vi "Write Command.vi"(7 "Addr":string, 10 "Input Value":dbl, 11 "TEC Cmd":T1) -> (2 "Divisor":i32, 3 "Cmd":string)   [LabVIEW 2018, in "TE Cooler.lvlib" / "TE Cooler.lvclass"]
uses:
  TE Cooler.lvclass
  Controls/Command.ctl
  Controls/Scale IO.ctl
  Controls/Hex Cmd.ctl
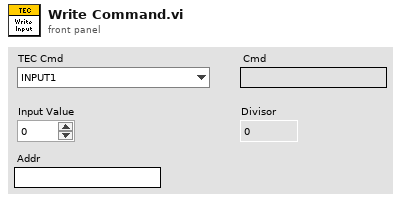
[diagram p1: front panel]
types:
  T1 = typedef "TE Cooler.lvlib/TE Cooler.lvclass/Command.ctl" = enum16{"INPUT1", "DESIRED CONTROL VALUE", "POWER OUTPUT", "ALARM STATUS", "INPUT 2", "OUTPUT CURRENT COUNTS", "ALARM TYPE", "SET TYPE DEFINE", "SENSOR TYPE", "CONTROL TYPE", "CONTROL OUTPUT POLARITY", "POWER ON/OFF", "OUTPUT SHUTDOWN IF ALARM", "FIXED DESIRED CONTROL SETTING", "PROPORTIONAL BANDWIDTH", "INTEGRAL GAIN", "DERIVATIVE GAIN", "LOW EXTERNAL SET RANGE", "HIGH EXTERNAL SET RANGE", "ALARM DEADBAND", "HIGH ALARM SETTING", "LOW ALARM SETTING", "CONTROL DEADBAND SETTING", "INPUT1 OFFSET", "INPUT2 OFFSET", "HEAT MULTIPLIER", "COOL MULTIPLIER", "OVER CURRENT COUNT COMPARE VALUE", "ALARM LATCH ENABLE", "NOT USED", "ALARM LATCH RESET", "CHOOSE SENSOR FOR ALARM FUNCTION", "CHOOSE TEMPERATURE WORKING UNITS", "EEPROM WRITE ENABLE", "OVER CURRENT CONTINUOUS", "OVER CURRENT RESTART ATTEMPTS", "JP3 DISPLAY ENABLE"}
  T2 = typedef "TE Cooler.lvlib/TE Cooler.lvclass/Hex Cmd.ctl" = string[][]
  T3 = typedef "TE Cooler.lvlib/TE Cooler.lvclass/Scale IO.ctl" = i32[][]
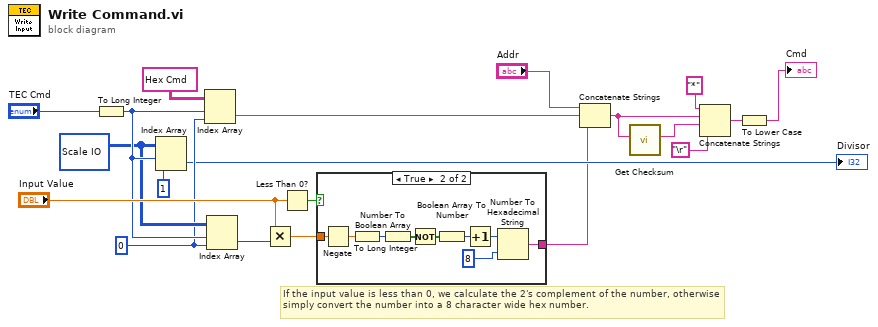
[diagram p0: block diagram]
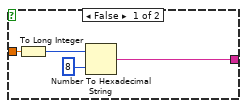
[diagram p2: hidden frame]
diagram:
  w15 = T3 [[0, 100], [0, 100], [0, 511], [0, 1], [0, 100], [0, 1], [1, 1], [1, 1], [1, 1], [1, 1], [1, 1], [1, 1], [100, 100], [100, 100], [100, 100], [100, 100], [1, 1], [1, 1], [100, 100], [100, 100], [100, 100], [100, 100], [100, 100], [100, 100], [100, 100], [100, 100], [100, 100], [1, 1], [1, 1], [0, 0], [1, 0], [1, 1], [1, 1], [1, 1], [1, 1], [1, 1], [1, 1]] ("Scale IO")
  w14 = 0 ("index (col)")
  # "If the input value is less than 0, we calculate the 2's complement of the number, otherwise simply convert the number into a 8 character wide hex number."
  n1 = To Long Integer(number="TEC Cmd") -> (32bit integer=w19:i32)
  n2 = Index Array(array=w15, index (row)=w19, index (col)=1 ("disabled index (col)")) -> (element=→"Divisor":i32)
  n3 = Index Array(array=T2 [["", "01"], ["", "03"], ["", "02"], ["", "05"], ["", "06"], ["", "07"], ["28", "41"], ["29", "42"], ["2a", "43"], ["2b", "44"], ["2c", "45"], ["2d", "46"], ["2e", "47"], ["1c", "50"], ["1d", "51"], ["1e", "52"], ["1f", "53"], ["20", "54"], ["21", "55"], ["22", "56"], ["23", "57"], ["24", "58"], ["25", "59"], ["26", "5a"], ["27", "5b"], ["0c", "5c"], ["0d", "5d"], ["0e", "5e"], ["2f", "48"], ["", ""], ["33", ""], ["31", "4a"], ["32", "4b"], ["34", "4c"], ["35", "4d"], ["0f", "5f"], ["36", "4e"]] ("Hex Cmd"), index (row)=w19, index (col)=w14) -> (element=w7:string)
  n4 = Index Array(array=w15, index (row)=w19, index (col)=w14) -> (element=w8:i32)
  n5 = Multiply(x="Input Value", y=w8) -> (x*y=w13:dbl)
  n6 = Less Than 0?(x="Input Value") -> (x < 0?=w12:bool)
  n7 = case shown="True" w12 {
    tunnel: [w23 w29] -> w2
    tunnel: w13 -> [w22 w25]
    frame False {
      n8 = To Long Integer(number=w22) -> (32bit integer=w21:i32)
      n9 = Number To Hexadecimal String(1:i16 8 ("width (-)"), 2:w21) -> (0:w23:string)
    }
    frame True {
      n10 = Negate(x=w25) -> (-x=w26:dbl)
      n11 = To Long Integer(number=w26) -> (32bit integer=w27:i32)
      n12 = Number To Boolean Array(number=w27) -> (Boolean array=w33:bool[])
      n13 = Not(x=w33) -> (.not. x?=w32:bool[])
      n14 = Boolean Array To Number(Boolean array=w32) -> (number=w31:u32)
      n15 = Increment(x=w31) -> (x+1=w28:u32)
      n16 = Number To Hexadecimal String(1:i16 8 ("width (-)"), 2:w28) -> (0:w29:string)
    }
  }
  n17 = Concatenate Strings("Addr", w7, w2) -> (w4:string)
  n18 = call "Get Checksum.vi"("Input"=w4) -> ("Checksum"=w5:string)  [unwired: 10 in]
  n19 = Concatenate Strings("*" ("string"), w4, w5, "\r" ("string")) -> (w11:string)
  n20 = To Lower Case(string=w11) -> (all lower case string=→"Cmd":string)
